vi "User Interface.vi"(11 "Sequencer in":refnum<class "Sequencer.lvclass">) -> ()   [LabVIEW 2024, in "Ramses Sequencer.lvlib" / "Sequencer.lvclass"]
uses:
  Sequencer.lvclass
  <vilib>/Utility/miscctls.llb/LVRowAndColumnUnsignedTypeDef.ctl
panel:
  out "Test Steps":i32(listbox)
  in  "Close":bool
  out "Status":string
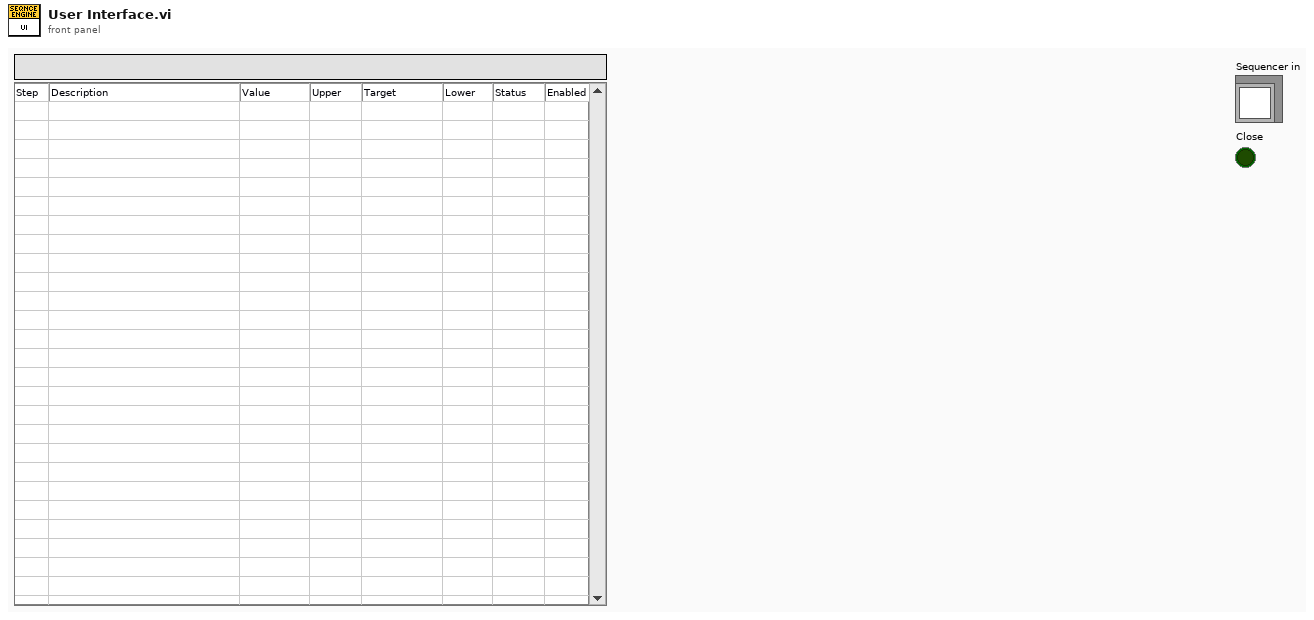
[diagram p1: front panel]
types:
  T1 = typedef "LVRowAndColumnUnsignedTypeDef.ctl" = cluster{"Row":u32, "Column":u32}
  T2 = typedef "Ramses Sequencer.lvlib/Sequencer.lvclass/Sequencer State -- enum.ctl" = enum16{"Idle", "Running", "Paused", "Complete"}
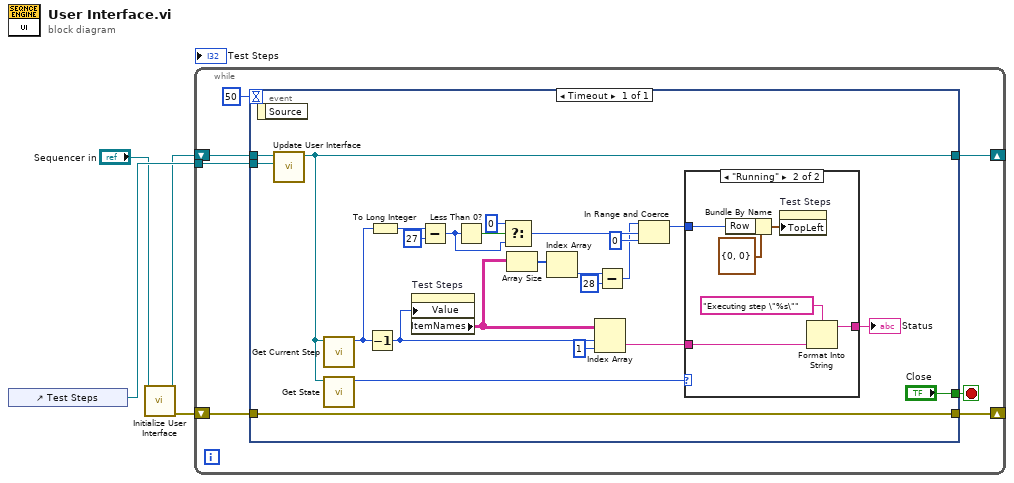
[diagram p0: block diagram]
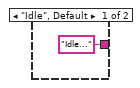
[diagram p2: hidden frame]
diagram:
  n1 = control-ref of="Test Steps"() -> (w4:refnum<vi>)
  n2 = call "Initialize User Interface.vi"("Sequencer in"="Sequencer in") -> ("error out"=w1:errorcluster, "Sequencer out"=w2:refnum<class "Sequencer.lvclass">)  [unwired: 9 in]
  n3 = while {
    shift-right: [w10] -> _
    shift-left: w2 -> [w11]
    shift-right: [w8] -> _
    shift-left: w1 -> [w9]
    tunnel: w4 -> [w5]
    stop <- w6 stop-if-true
    n4 = event shown="[0] Timeout" {
      selector: _ -> [_]
      dyn-events: _ -> [_]
      timeout: 50 -> [_]
      tunnel: w11 -> [w14]
      tunnel: [w13] -> w10
      tunnel: w9 -> [w35]
      tunnel: [w35] -> w8
      tunnel: ["Close"] -> w6
      tunnel: w5 -> [w12]
      event Timeout {
        n5 = event-data() -> ()  [unwired: 1 in, 1 out]
        n6 = call "Update User Interface.vi"("Refnum"=w12, "Sequencer in"=w14) -> ("Sequencer out"=w13:refnum<class "Sequencer.lvclass">)  [unwired: 8 in, 1 out]
        n7 = call "Get Current Step.vi"("Sequencer in"=w13) -> ("Current Step"=w28:u32)  [unwired: 9 in, 1 out]
        n8 = call "Get State.vi"("Sequencer in"=w13) -> ("Sequencer State"=w34:T2)  [unwired: 9 in, 1 out]
        n9 = Decrement(x=w28) -> (x-1=w29:u32)
        n10 = To Long Integer(number=w28) -> (32bit integer=w22:i32)
        n11 = property on="Test Steps" class="MCListbox (strict)"("Value"=w29) -> ("ItemNames"=w27:string[][])  [unwired: 2 in, 2 out]
        n12 = Subtract(x=w22, y=27) -> (x-y=w17:i32)
        n13 = Less Than 0?(x=w17) -> (x < 0?=w20:bool)
        n14 = Select(t=u32 0 ("upper limit"), s=w20, f=w17) -> (s? t:f=w18:u32)
        n15 = Array Size(array=w27) -> (size(s)=w26:i32[])
        n16 = Index Array(array=w26) -> (element=w25:i32)  [unwired: 1 in]
        n17 = Index Array(array=w27, index (row)=w29, index (col)=1 ("disabled index (col)")) -> (element=w30:string)
        n18 = Subtract(x=w25, y=28) -> (x-y=w16:i32)
        n19 = In Range and Coerce(upper limit=w16, x=w18, lower limit=u32 0 ("upper limit")) -> (coerced(x)=w15:u32)  [unwired: 1 out]
        n20 = case shown="\"Running\"" w34 {
          tunnel: ["Idle..." w41] -> w33
          tunnel: w30 -> [_ w40]
          tunnel: w15 -> [_ w37]
          frame "Idle", Default {
          }
          frame "Running" {
            n21 = Bundle By Name(cluster=T1 {"Row"=0, "Column"=0} ("Top Left Visible Cell"), "Row"=w37) -> (w39:T1)
            n22 = property on="Test Steps" class="MCListbox (strict)"("TopLeft"=w39) -> ()  [unwired: 2 in, 2 out]
            n23 = Format Into String(format string="Executing step \"%s\"", w40) -> (resulting string=w41:string)  [unwired: 2 in, 1 out]
          }
        }
        "Status" <- w33
      }
    }
  }
